vi "Open.vi"(8 "error in (no error)":errorcluster, 10 "address":string, 11 "Instrument.SR7270 in":refnum<class "Instrument.SR7270.lvclass">) -> (0 "error out":errorcluster, 3 "Instrument.SR7270 out":refnum<class "Instrument.SR7270.lvclass">)   [LabVIEW 2019, in "Instrument.SR7270.lvclass"]
uses:
  Instrument.SR7270.lvclass
  <userlib>/LevyLab/Instrument Framework/SMOs/Instrument/Instrument.lvclass
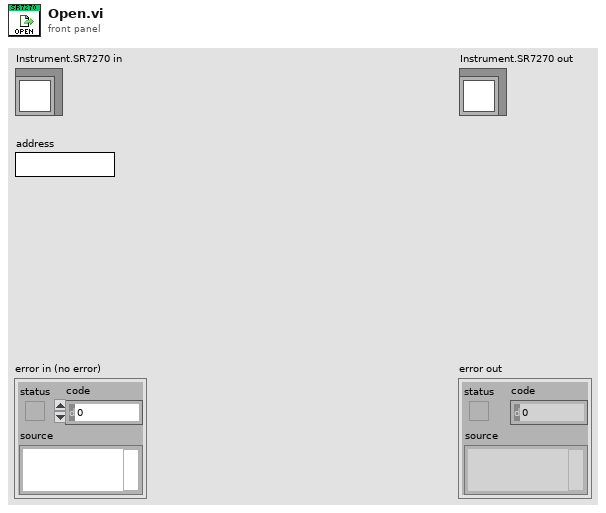
[diagram p1: front panel]
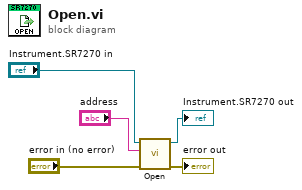
[diagram p0: block diagram]
diagram:
  n1 = call-parent "Open.vi"("error in (no error)"="error in (no error)", "address"="address", "Instrument in"="Instrument.SR7270 in") -> ("error out"=→"error out":errorcluster, "Instrument out"=→"Instrument.SR7270 out":refnum<class "Instrument.SR7270.lvclass">)  [unwired: 7 in]
